vi "EncoderOffset.vi"(10 "Numeric in":dbl, 11 "Set?":bool) -> (2 "Numeric out":dbl)   [LabVIEW 2013]
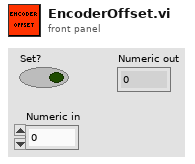
[diagram p1: front panel]
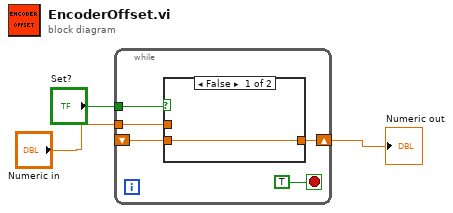
[diagram p0: block diagram]
diagram:
  n1 = while {
    tunnel: "Set?" -> [w7]
    shift-right: [w5] -> w3
    shift-left: _ -> [w6]
    tunnel: "Numeric in" -> [w4]
    stop <- TRUE stop-if-true
    n2 = case shown="False" w7 {
      tunnel: w6 -> [w9 _]
      tunnel: [w9 w10] -> w5
      tunnel: w4 -> [_ w10]
      frame False {
      }
      frame True {
      }
    }
  }
  "Numeric out" <- w3
